vi "LINX - Interactions Seven Segement Display.vi"() -> ()   [LabVIEW 2011]
doc: "This example demonstrates how to use the Seven Segment display from the Digilent Interactions Kit with LINX custom commands and periodic tasks."
uses:
  vi.lib/MakerHub/LINX/Public/Utilities/Open Serial.vi
  vi.lib/MakerHub/LINX/LMH-LINX.lvlib
  vi.lib/MakerHub/LINX/Public/Sensors/Digilent/Interaction Parts Kit/Interaction Parts Kit.lvlib
panel:
  in  "Channels":T1
  in  "Value To Display":u16
  in  "Display Type":enum8{"Matrix", "7 Segment"}(ring)=enum."7 Segment"
  in  "Smart Write? (T)":bool=TRUE
  out "Loop Rate (Hz)":u32
  in  "Stop Button":bool
  in  "Serial Port":refnum<visa-resource-name>="N/A"
  # "Seven Segment Display\n\nThis example demonstrates how to use the seven segment display included in the LabVIEW Interactions Parts Kit.  \nMake sure that you are using the correct firmware version so the matrix functions are supported. \n\nInstructions:\n1. Select the COM Port associated with the LINX device\n2. Toggle the Smart Write to desired value\n3. Enter the 12 Channels connected to seven segment display in the correct order (enter 0 for pins 13-16)\n4. Enter \"7 Segment\" under Display Type\n5. Click the Run Arrow."
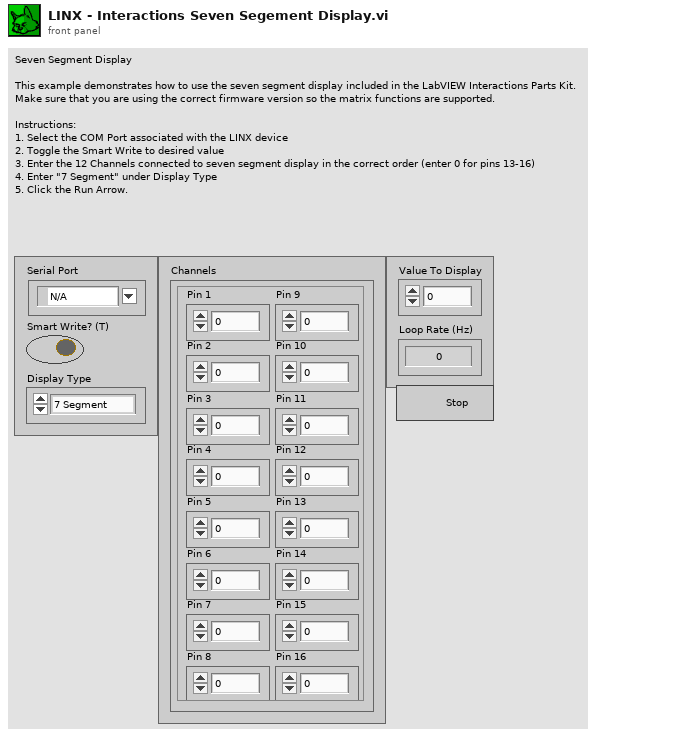
[diagram p1: front panel]
types:
  T1 = cluster{"Pin 1":u8, "Pin 2":u8, "Pin 3":u8, "Pin 4":u8, "Pin 5":u8, "Pin 6":u8, "Pin 7":u8, "Pin 8":u8, "Pin 9":u8, "Pin 10":u8, "Pin 11":u8, "Pin 12":u8, "Pin 13":u8, "Pin 14":u8, "Pin 15":u8, "Pin 16":u8}
  T2 = typedef "LMH-LINX.lvlib/LINX Ref.ctl" = cluster{"IO":T3, "Interface":T4, "LINX Device Config":T5}
  T3 = typedef "LMH-LINX.lvlib/Platform.ctl" = enum16{"Remote", "Local"}
  T4 = typedef "LMH-LINX.lvlib/Interface.ctl" = enum16{"Serial", "TCP"}
  T5 = typedef "LMH-LINX.lvlib/Device.lvlib/LINX Device Config.ctl" = cluster{"Interface":T4, "COM Port":refnum<visa-resource-name>, "TCP Configuration":T6, "Device Family":u8, "Device ID":u8, "Device Name":string, "TCP Ref":refnum<k5>, "Channels":T7}
  T6 = typedef "LMH-LINX.lvlib/Device.lvlib/TCP Config.ctl" = cluster{"IP Address":string, "Port":u16}
  T7 = typedef "LMH-LINX.lvlib/Channels.ctl" = cluster{"DI":u8[], "DO":u8[], "AI":u8[], "AO":u8[], "PWM":u8[], "QE":u8[], "UART":u8[], "I2C 2":u8[], "SPI":u8[], "CAN":u8[], "Servo":u8[], "AI Ref (V)":dbl, "AI Resolution (Bits)":u8, "AO Ref (V)":dbl, "AO Resolution (Bits)":u8}
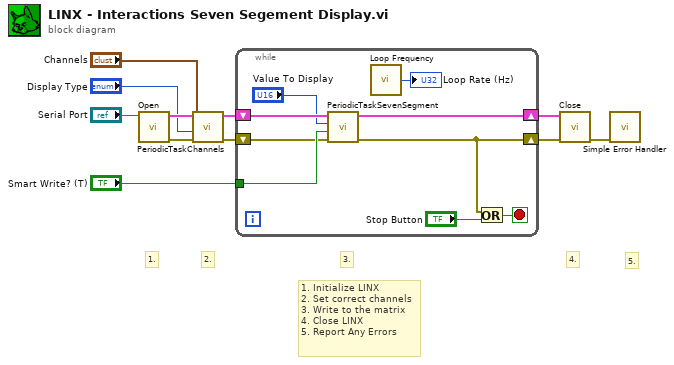
[diagram p0: block diagram]
diagram:
  # "5."
  # "1."
  # "2."
  # "3."
  # "4."
  # "1. Initialize LINX\n2. Set correct channels\n3. Write to the matrix\n4. Close LINX\n5. Report Any Errors"
  n1 = call-poly "Open.vi"("Serial Port"="Serial Port") -> ("Error Out"=w9:errorcluster, "LINX Resource"=w10:T2)  [unwired: 8 in, 1 out]
  n2 = call "PeriodicTaskChannels.vi"("Error In"=w9, "Display Type"="Display Type", "Channels"="Channels", "LINX Resource"=w10) -> ("Error Out"=w8:errorcluster, "LINX Resource"=w7:T2)  [unwired: 4 in, 1 out]
  n3 = while {
    shift-right: [w13] -> w5
    shift-left: w8 -> [w17]
    shift-right: [w20] -> w6
    shift-left: w7 -> [w16]
    tunnel: "Smart Write? (T)" -> [w18]
    stop <- w14 stop-if-true
    n4 = call "PeriodicTaskSevenSegment.vi"("Error In"=w17, "Smart Write? (T)"=w18, "Value To Display"="Value To Display", "LINX Resource"=w16) -> ("Error Out"=w13:errorcluster, "LINX Resource"=w20:T2)  [unwired: 5 in, 1 out]
    n5 = call "Loop Frequency.vi"() -> ("Loop Rate (Hz)"=→"Loop Rate (Hz)":u32)
    n6 = Or(x=w13, y="Stop Button") -> (x .or. y?=w14:bool)
  }
  n7 = call "Close.vi"("Error In"=w5, "LINX Resource"=w6) -> ("Error Out"=w1:errorcluster)  [unwired: 9 in]
  n8 = call <vilib>:"Simple Error Handler.vi"("error in (no error)"=w1) -> ()  [unwired: 4 in, 5 out]
